vi "Labspec LoadAll.vi"(8 "error in":errorcluster, 9 "Path":path, 11 "Automation Refnum In":refnum<k7>) -> (0 "error out":errorcluster, 1 "DataID":i32[](array[numeric]), 3 "Automation Refnum Out":refnum<k7>)   [LabVIEW 2014]
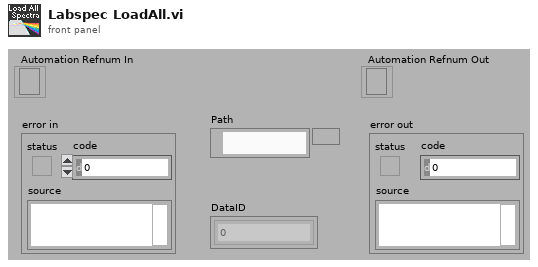
[diagram p1: front panel]
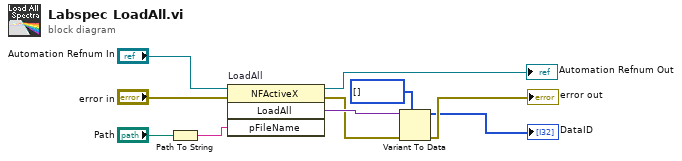
[diagram p0: block diagram]
diagram:
  n1 = Path To String(path="Path") -> (string=w8:string)
  n2 = invoke on="LoadAll" class="NFActiveX" method="LoadAll"(reference="Automation Refnum In", error in="error in", "pFileName"=w8) -> (reference out=→"Automation Refnum Out":refnum<k7>, error out=w4:errorcluster, "LoadAll"=w5:variant)  [unwired: 1 in, 1 out]
  n3 = Variant To Data(error in=w4, type=i32[] [] ("Array"), Variant=w5) -> (data=→"DataID":i32[], error out=→"error out":errorcluster)
